vi "AutoAlign_P612_Oct8th2015.vi"() -> ()   [LabVIEW 2014]
uses:
  Controls/GraphNotifier2D.ctl
  Controls/StageStates.ctl
panel:
  out "Aligned":bool
  in  "Repeat":bool
  in  "Start":bool
  out "Intensity Graph":sgl[][](graph)
  in  "Quit":bool
  out "Sample":cluster{"X":dbl, "Y":dbl}[](graph)
  in  "Accumulations":i32=10
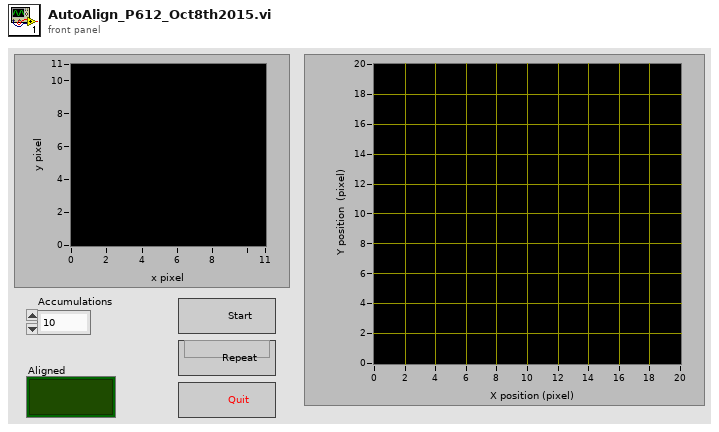
[diagram p1: front panel]
types:
  T1 = typedef "GraphNotifier2D.ctl" = cluster{"Xpos":i32, "Ypos":i32, "subarray":sgl[][], "Intensity":sgl}
  T2 = typedef "LabVIEW Interface for Arduino.lvlib/Arduino Resource.ctl" = cluster{"VISA resource":refnum<visa-resource-name>, "Board Type":T3, "Connection Type":enum8{"USB / Serial"}, "Bytes Per Packet (15)":u8}
  T3 = typedef "LabVIEW Interface for Arduino.lvlib/Board Type.ctl" = enum16{"Uno", "Dimuelanove w/Atmega 328", "Mega 2560"}
  T4 = typedef "StageStates.ctl" = enum16{"POSITION", "MVR", "MOVE", "HALT", "ONTARGET", "ERROR", "EXIT", "HOME", "ZEROPOS", "NANOPOS", "QUIT", "ANALOG"}
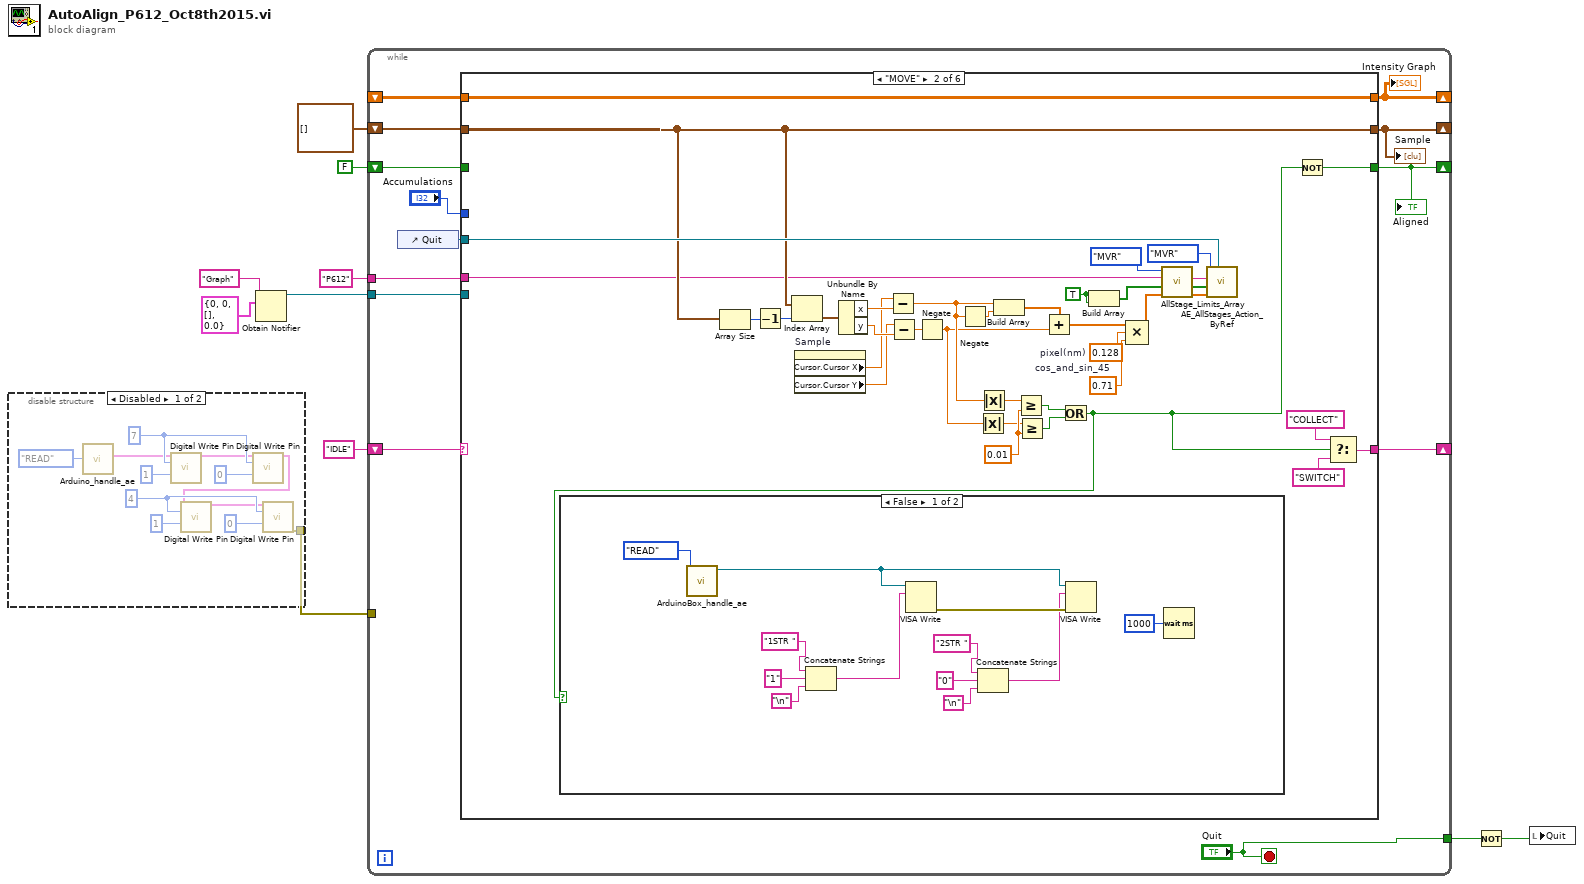
[diagram p0: block diagram]
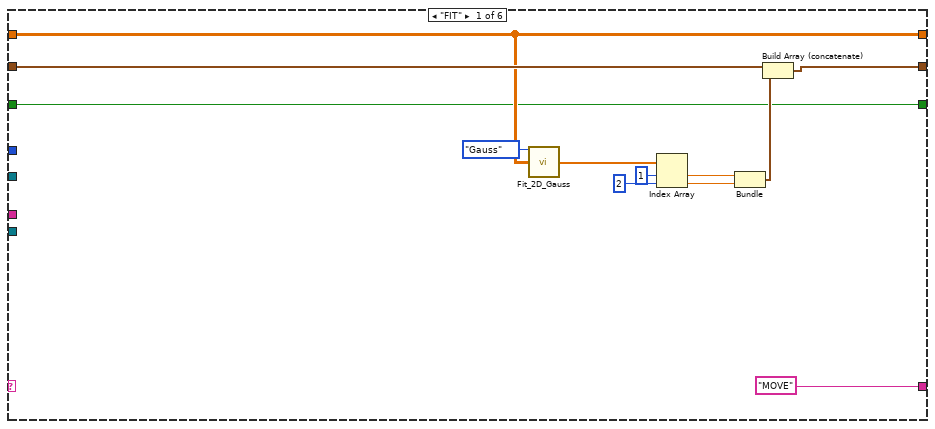
[diagram p3: hidden frame]
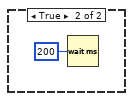
[diagram p4: hidden frame]
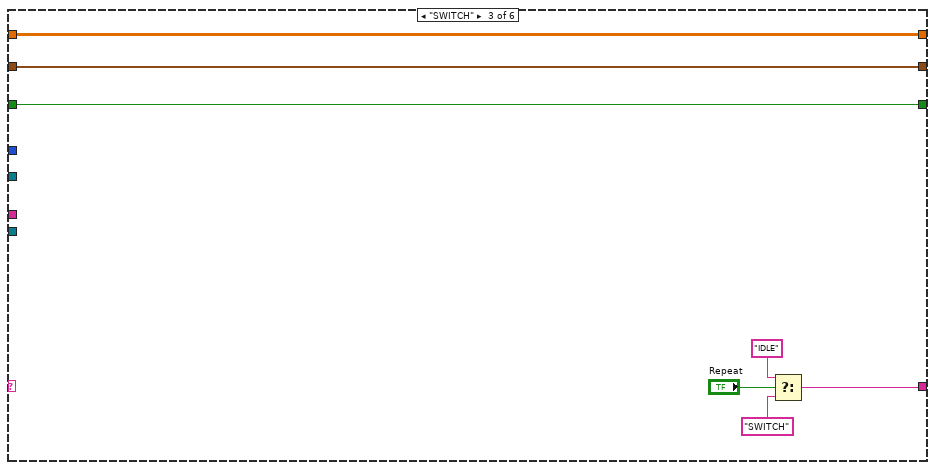
[diagram p5: hidden frame]
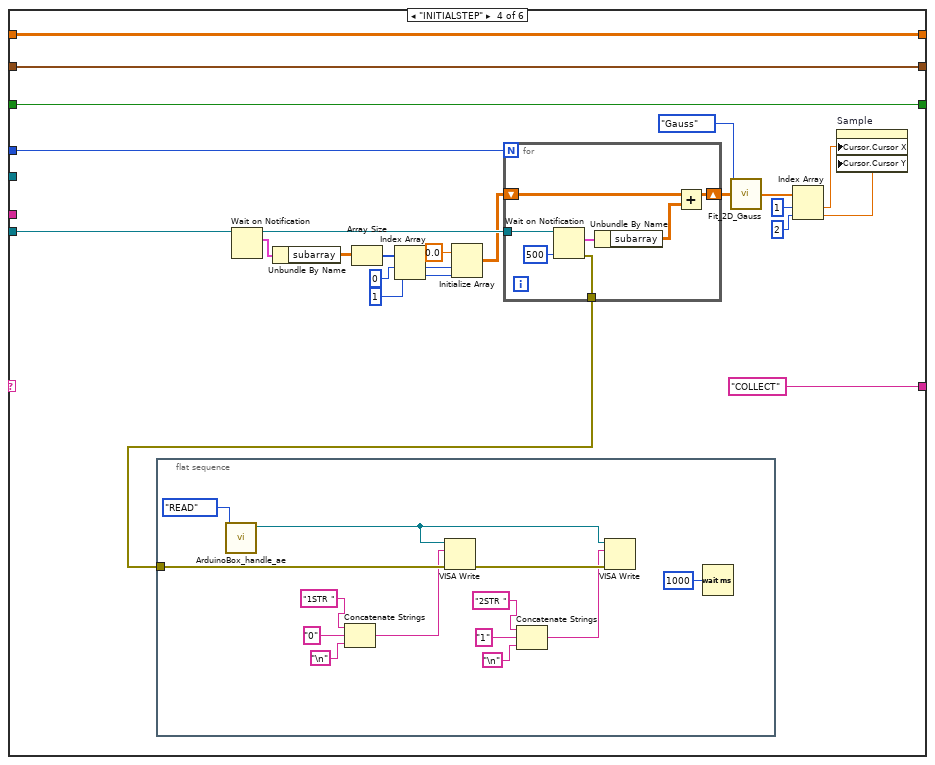
[diagram p6: hidden frame]
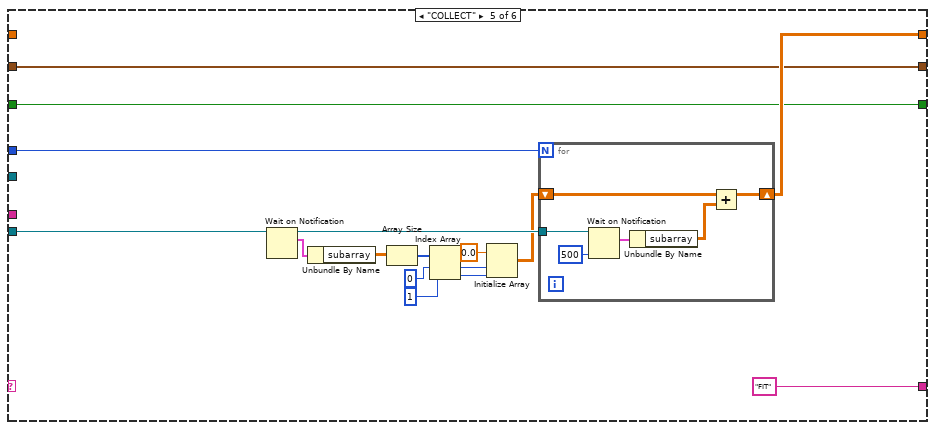
[diagram p7: hidden frame]
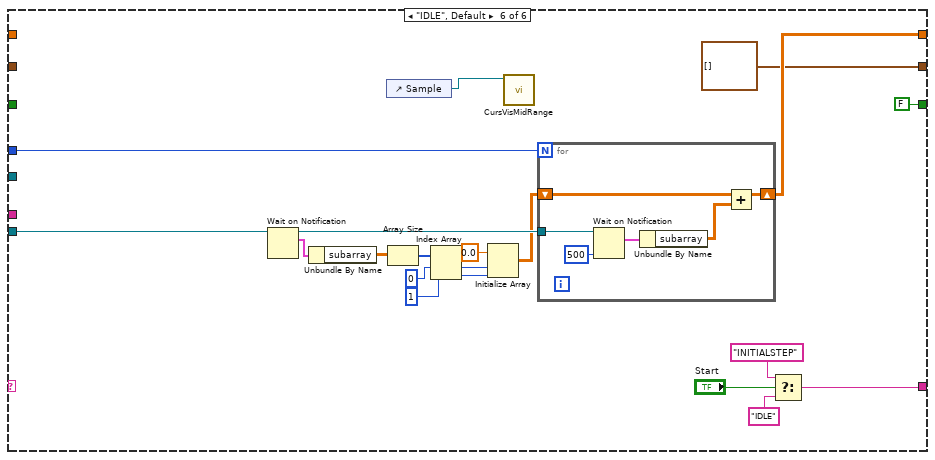
[diagram p8: hidden frame]
diagram:
  n1 = disable-structure shown="Disabled" {
    disable-tunnel: [w11 _] -> w6
    frame Disabled {
      w22 = u8 4 ("Digital I/O Pin (0)")
      w17 = u8 7 ("Digital I/O Pin (0)")
      n2 = call "Arduino_handle_ae.vi"("Enum"=enum16{"WRITE", "READ"}."READ") -> ("Arduino Resource Out"=w16:T2)  [unwired: 10 in]
      n3 = call <vilib>:"Digital Write Pin.vi"("Arduino Resource"=w16, "Digital I/O Pin (0)"=w17, "Value (0)"=u8 1) -> ("Arduino Resource"=w12:T2)  [unwired: 11 in, 1 out]
      n4 = call <vilib>:"Digital Write Pin.vi"("Arduino Resource"=w12, "Digital I/O Pin (0)"=w17, "Value (0)"=u8 0) -> ("Arduino Resource"=w21:T2)  [unwired: 11 in, 1 out]
      n5 = call <vilib>:"Digital Write Pin.vi"("Arduino Resource"=w21, "Digital I/O Pin (0)"=w22, "Value (0)"=u8 1) -> ("Arduino Resource"=w20:T2)  [unwired: 11 in, 1 out]
      n6 = call <vilib>:"Digital Write Pin.vi"("Arduino Resource"=w20, "Digital I/O Pin (0)"=w22, "Value (0)"=u8 0) -> ("error out"=w11:errorcluster)  [unwired: 11 in, 1 out]
    }
    frame Enabled {
    }
  }
  n7 = Obtain Notifier(name (unnamed)="Graph", notification data type=T1 {"Xpos"=0, "Ypos"=0, "subarray"=[], "Intensity"=0.0}) -> (notifier out=w3:refnum<notifier>)  [unwired: 2 in, 2 out]
  n8 = while {
    shift-right: [w33] -> _
    shift-left: _ -> [w35]
    shift-right: [w34] -> _
    shift-left: cluster{"x":dbl, "y":dbl}[] [] ("XY chart data") -> [w24]
    shift-right: [w32] -> _
    shift-left: "IDLE" -> [w28]
    shift-right: [w30] -> _
    shift-left: FALSE -> [w31]
    tunnel: w3 -> [w27]
    tunnel: "P612" ("StageID") -> [w25]
    tunnel: w6 -> [_]
    tunnel: ["Quit"] -> w2
    stop <- "Quit" stop-if-true
    n9 = control-ref of="Quit"() -> (w29:refnum<vi>)
    n10 = case shown="\"MOVE\"" w28 {
      tunnel: [w43 w84 w102 w128 w164 w190] -> w33
      tunnel: w35 -> [w43 w84 w102 w128 _ _]
      tunnel: w24 -> [w45 w57 w103 w125 w163 _]
      tunnel: [w44 w57 w103 w125 w163 cluster{"x":dbl, "y":dbl}[] [] ("XY chart data")] -> w34
      tunnel: w25 -> [_ w51 _ _ _ _]
      tunnel: ["MOVE" w70 w99 "COLLECT" "FIT" w188] -> w32
      tunnel: w31 -> [w41 _ w104 w127 w162 _]
      tunnel: [w41 w56 w104 w127 w162 FALSE] -> w30
      tunnel: w29 -> [_ w75 _ _ _ _]
      tunnel: w27 -> [_ _ _ w113 w151 w181]
      tunnel: "Accumulations" -> [_ _ _ w114 w160 w185]
      frame "FIT" {
        n11 = call "Fit_2D_Gauss.vi"("Enum"=enum16{"Gauss", "Lorentz"}."Gauss", "Image IN"=w43) -> ("Fit Parameters"=w47:dbl[])  [unwired: 12 in, 1 out]
        n12 = Index Array(array=w47, index #1=1 ("index"), index #2=2 ("index")) -> (element #1=w38:dbl, element #2=w37:dbl)
        n13 = Bundle("Numeric"=w38, "Numeric"=w37) -> (w46:cluster{"Numeric":dbl, "Numeric":dbl})  [unwired: 1 in]
        n14 = Build Array (concatenate)(w45, w46) -> (w44:cluster{"Numeric":dbl, "Numeric":dbl}[])
      }
      frame "MOVE" {
        w69 = 0.71  # cos_and_sin_45
        w83 = 0.01 ("y")
        w82 = 0.128  # pixel(nm)
        w81 = TRUE
        n15 = Array Size(array=w57) -> (size(s)=w76:i32)
        n16 = Decrement(x=w76) -> (x-1=w68:i32)
        n17 = Index Array(array=w57, index=w68) -> (element=w77:cluster{"x":dbl, "y":dbl})
        n18 = property on="Sample" class="XYGraph (strict)"() -> ("Cursor.Cursor X"=w74:dbl, "Cursor.Cursor Y"=w73:dbl)  [unwired: 2 in, 2 out]
        n19 = Unbundle By Name(w77) -> ("x"=w78:dbl, "y"=w79:dbl)
        n20 = Subtract(x=w74, y=w78) -> (x-y=w64:dbl)
        n21 = Subtract(x=w73, y=w79) -> (x-y=w65:dbl)
        n22 = Negate(x=w65) -> (-x=w61:dbl)
        n23 = Negate(x=w64) -> (-x=w63:dbl)
        n24 = Absolute Value(x=w61) -> (abs(x)=w66:dbl)
        n25 = Absolute Value(x=w64) -> (abs(x)=w67:dbl)
        n26 = Build Array(w64, w63) -> (w62:dbl[])
        n27 = Greater Or Equal?(x=w67, y=w83) -> (x >= y?=w59:bool)
        n28 = Greater Or Equal?(x=w66, y=w83) -> (x >= y?=w58:bool)
        n29 = Add(x=w62, y=w61) -> (x+y=w60:dbl[])
        n30 = Or(x=w59, y=w58) -> (x .or. y?=w48:bool)
        n31 = case shown="False" w48 {
          frame False {
            n32 = call "ArduinoBox_handle_ae.vi"("Enum"=enum16{"WRITE", "READ"}."READ") -> ("VISA resource Out"=w90:refnum<visa-resource-name>)  [unwired: 10 in]
            n33 = Concatenate Strings("1STR ", "1" ("string"), "\n") -> (w93:string)
            n34 = VISA Write(VISA resource name=w90, write buffer=w93) -> (error out=w91:errorcluster)  [unwired: 1 in, 2 out]
            n35 = Concatenate Strings("2STR ", "0" ("string"), "\n") -> (w86:string)
            n36 = VISA Write(VISA resource name=w90, write buffer=w86, error in (no error)=w91) -> ()  [unwired: 3 out]
            n37 = Wait (ms)(milliseconds to wait=u32 1000) -> ()  [unwired: 1 out]
          }
          frame True {
            n38 = Wait (ms)(milliseconds to wait=u32 200) -> ()  [unwired: 1 out]
          }
        }
        n39 = Build Array(w81, w81) -> (w50:bool[])
        n40 = Compound Arithmetic op=MULTIPLY(w60, w82, w69) -> (w52:dbl[])
        n41 = call "AllStage_Limits_Array.vi"("Step(um)/Position(units)"=w52, "Axis"=w50, "Stage ID"=w51, "MOVE/MVR"=enum16{"MOVE", "MVR"}."MVR") -> ("Positions"=w53:dbl[], "Boolean Array"=w54:bool[], "Stage ID"=w55:string)  [unwired: 5 in]
        n42 = call "AE_AllStages_Action_ByRef.vi"("Abort"=w75, "Positions"=w53, "Axis"=w54, "Stage ID"=w55, "Action"=StageStates."MVR") -> ()  [unwired: 3 in, 4 out]
        n43 = Not(x=w48) -> (.not. x?=w56:bool)
        n44 = Select(t="COLLECT", s=w48, f="SWITCH") -> (s? t:f=w70:string)
      }
      frame "SWITCH" {
        n45 = Select(t="IDLE", s="Repeat", f="SWITCH") -> (s? t:f=w99:string)
      }
      frame "INITIALSTEP" {
        n46 = flat-sequence {
          tunnel: w112 -> [w140]
          frame #0 {
            n47 = call "ArduinoBox_handle_ae.vi"("Enum"=enum16{"WRITE", "READ"}."READ") -> ("VISA resource Out"=w134:refnum<visa-resource-name>)  [unwired: 10 in]
            n48 = Concatenate Strings("1STR ", "0" ("string"), "\n") -> (w137:string)
            n49 = VISA Write(VISA resource name=w134, write buffer=w137, error in (no error)=w140) -> (error out=w135:errorcluster)  [unwired: 2 out]
            n50 = Concatenate Strings("2STR ", "1" ("string"), "\n") -> (w130:string)
            n51 = VISA Write(VISA resource name=w134, write buffer=w130, error in (no error)=w135) -> ()  [unwired: 3 out]
            n52 = Wait (ms)(milliseconds to wait=u32 1000) -> ()  [unwired: 1 out]
          }
        }
        n53 = Wait on Notification(notifier=w113) -> (notifier out=w116:refnum<notifier>, notification=w124:T1)  [unwired: 3 in, 2 out]
        n54 = Unbundle By Name(w124) -> ("subarray"=w123:sgl[][])
        n55 = Array Size(array=w123) -> (size(s)=w122:i32[])
        n56 = Index Array(array=w122, index #1=0 ("index"), index #2=1 ("index")) -> (element #1=w119:i32, element #2=w118:i32)
        n57 = Initialize Array(sgl 0.0 ("element"), w119, w118) -> (w115:sgl[][])
        n58 = for {
          N: w114 -> [_]
          shift-right: [w148] -> w108
          shift-left: w115 -> [w147]
          tunnel: w116 -> [w145]
          tunnel: [w142] -> w112
          n59 = Wait on Notification(notifier=w145, timeout in ms (-1)=500) -> (notification=w144:T1, error out=w142:errorcluster)  [unwired: 2 in, 2 out]
          n60 = Unbundle By Name(w144) -> ("subarray"=w143:sgl[][])
          n61 = Add(x=w147, y=w143) -> (x+y=w148:sgl[][])
        }
        n62 = call "Fit_2D_Gauss.vi"("Enum"=enum16{"Gauss", "Lorentz"}."Gauss", "Image IN"=w108) -> ("Fit Parameters"=w111:dbl[])  [unwired: 12 in, 1 out]
        n63 = Index Array(array=w111, index #1=1 ("index"), index #2=2 ("index")) -> (element #1=w107:dbl, element #2=w106:dbl)
        n64 = property on="Sample" class="XYGraph (strict)"("Cursor.Cursor X"=w107, "Cursor.Cursor Y"=w106) -> ()  [unwired: 2 in, 2 out]
      }
      frame "COLLECT" {
        n65 = Wait on Notification(notifier=w151) -> (notifier out=w150:refnum<notifier>, notification=w159:T1)  [unwired: 3 in, 2 out]
        n66 = Unbundle By Name(w159) -> ("subarray"=w158:sgl[][])
        n67 = Array Size(array=w158) -> (size(s)=w157:i32[])
        n68 = Index Array(array=w157, index #1=0 ("index"), index #2=1 ("index")) -> (element #1=w154:i32, element #2=w153:i32)
        n69 = Initialize Array(sgl 0.0 ("element"), w154, w153) -> (w149:sgl[][])
        n70 = for {
          N: w160 -> [_]
          shift-right: [w170] -> w164
          shift-left: w149 -> [w169]
          tunnel: w150 -> [w167]
          n71 = Wait on Notification(notifier=w167, timeout in ms (-1)=500) -> (notification=w166:T1)  [unwired: 2 in, 3 out]
          n72 = Unbundle By Name(w166) -> ("subarray"=w165:sgl[][])
          n73 = Add(x=w169, y=w165) -> (x+y=w170:sgl[][])
        }
      }
      frame "IDLE", Default {
        n74 = Wait on Notification(notifier=w181) -> (notifier out=w180:refnum<notifier>, notification=w183:T1)  [unwired: 3 in, 2 out]
        n75 = Unbundle By Name(w183) -> ("subarray"=w182:sgl[][])
        n76 = control-ref of="Sample"() -> (w172:refnum<vi>)
        n77 = Array Size(array=w182) -> (size(s)=w179:i32[])
        n78 = Index Array(array=w179, index #1=0 ("index"), index #2=1 ("index")) -> (element #1=w176:i32, element #2=w175:i32)
        n79 = Initialize Array(sgl 0.0 ("element"), w176, w175) -> (w173:sgl[][])
        n80 = call "CursVisMidRange.vi"("XYGraph in"=w172) -> ()  [unwired: 11 in]
        n81 = for {
          N: w185 -> [_]
          shift-right: [w196] -> w190
          shift-left: w173 -> [w195]
          tunnel: w180 -> [w193]
          n82 = Wait on Notification(notifier=w193, timeout in ms (-1)=500) -> (notification=w192:T1)  [unwired: 2 in, 3 out]
          n83 = Unbundle By Name(w192) -> ("subarray"=w191:sgl[][])
          n84 = Add(x=w195, y=w191) -> (x+y=w196:sgl[][])
        }
        n85 = Select(t="INITIALSTEP", s="Start", f="IDLE") -> (s? t:f=w188:string)
      }
    }
    "Sample" <- w34
    "Intensity Graph" <- w33
    "Aligned" <- w30
  }
  n86 = Not(x=w2) -> (.not. x?=w1:bool)
  n87 = local write "Quit"(w1) -> ()
